vi "Untitled 2.vi"() -> ()   [LabVIEW 2015]
panel:
  in  "Enum":T1(ring)
  in  "stop":bool
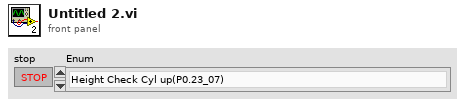
[diagram p1: front panel]
types:
  T1 = enum16{"Height Check Cyl up(P0.23_07)", "Height Check Cyl  Up RS_(AI12_26)", "Height Check Cyl  Dn RS_(AI13_27)", "Height Check Cyl dn(P0.24_08)", "Camera Cyl Rev(P0.26_10)", "Camera Cyl fwd(P0.25_09)", "Height Check Cyl off", "Camera Cyl Rev_RS(AI15_29)", "Camera Cyl off", "Camera Cyl FWD_RS(AI14_28)", "LCD Rotation Dn(P0.28_12)", "LCD Rotation dn proxi(AI17_31)", "LCD Rotation Up(P0.27_11)", "LCD Rotation dn proxi(AI16_30)"}
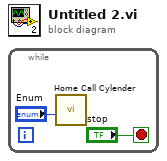
[diagram p0: block diagram]
diagram:
  n1 = while {
    stop <- "stop" stop-if-true
    n2 = call "Home Call Cylender.vi"("Enum"="Enum") -> ()  [unwired: 11 in]
  }
